vi "JetStages_GUI.vi"(10 "stop 2":refnum<vi>, 11 "GUI_cluster":T1={"Sub Panel"=refnum, "GUIdevice"="Bella_LP_Mode", "CtlRef"=refnum, "User Event in"=refnum}) -> ()   [LabVIEW 2020]
uses:
  Shared/GUI_Template/GUI_master/tcp new data cluster.ctl
  Controls/eventtypdef1.ctl
  Shared/GUI_Template/GUI_master/tcp_new_data_event.ctl
  Controls/GUI_cluster.ctl
panel:
  in  "stepsize::1":dbl=0.02 caption="stepsize" min=0.001 max=1.0
  in  "relativeMove.Axis 2neg::1":bool caption="+Y"
  in  "relativeMove.Axis 1neg::1":bool caption="-X"
  in  "relativeMove.Axis 2pos::1":bool caption="-Y"
  in  "relativeMove.Axis 1pos::1":bool caption="+X"
  in  "relativeMove.Axis 3neg::1":bool caption="-Z"
  in  "relativeMove.Axis 3pos::1":bool caption="+Z"
  in  "Status.Axis 3::1":u16(ring)=3 caption="Status" items=["Not referenced", "Homing", "Moving", "Ready"]
  in  "Position.Axis 3::1":dbl caption="Z" min=-12.0 max=12.0 format="%_4f"
  in  "Status.Axis 2::1":u16(ring)=3 caption="Status" items=["Not referenced", "Homing", "Moving", "Ready"]
  in  "Status.Axis 1::1":u16(ring)=3 items=["Not referenced", "Homing", "Moving", "Ready"]
  in  "Position.Axis 2::1":dbl caption="Y" min=-12.0 max=12.0 format="%_4f"
  in  "Position.Axis 1::1":dbl caption="X" min=-12.0 max=12.0 format="%_4f"
  in  "stop":bool
  out "tcp data event":T2
  out "GUIdevice 1":string="StagingHexapodPI"
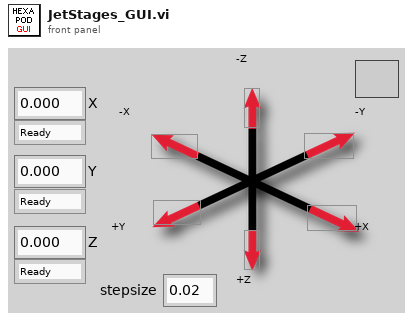
[diagram p1: front panel]
types:
  T1 = typedef "GUI_cluster.ctl" = cluster{"Sub Panel":refnum<vi>, "GUIdevice":string, "CtlRef":refnum<vi>, "User Event in":refnum<user-event>}
  T2 = typedef "tcp_new_data_event.ctl" = refnum<user-event>
  T3 = typedef "eventtypdef1.ctl" = cluster{"label":string, "Sub Panel":refnum<vi>, "CtlRef":refnum<vi>, "This VI":refnum<vi>}
  T4 = typedef "tcp new data cluster.ctl" = cluster{"EventEnum":enum16{"new data", "connection status update"}, "Device name":string}
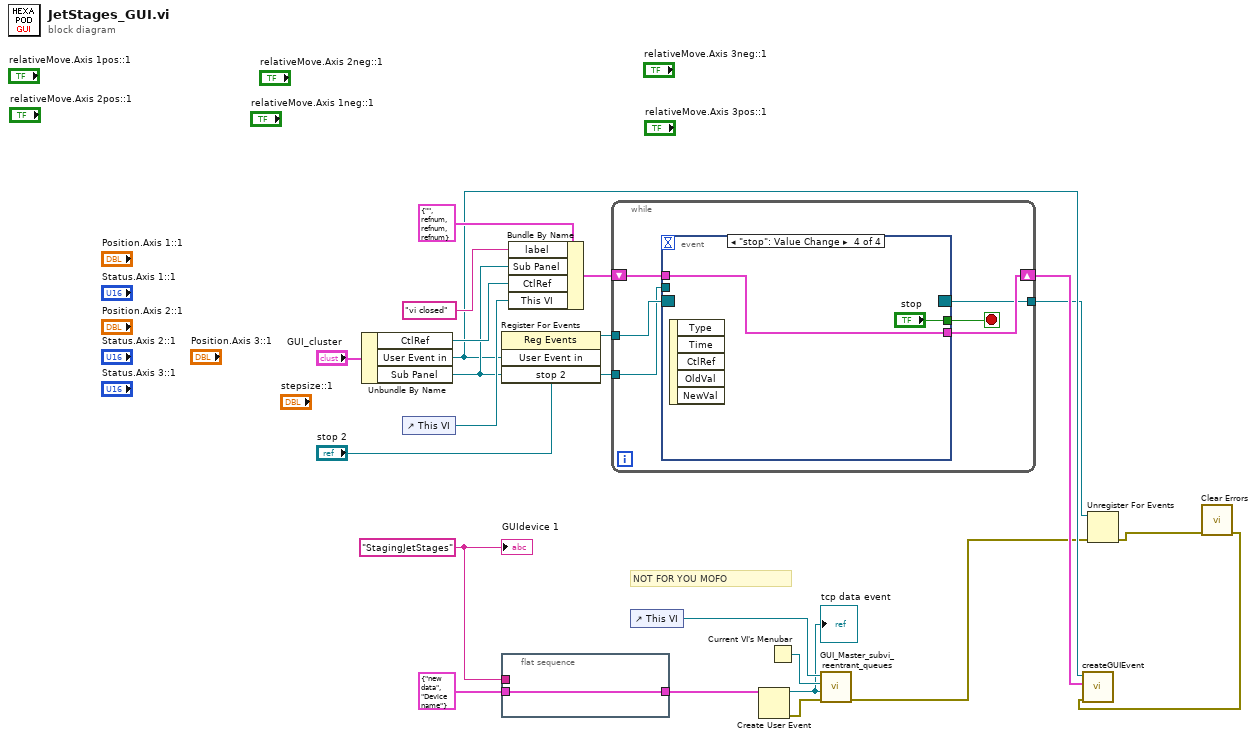
[diagram p0: block diagram]
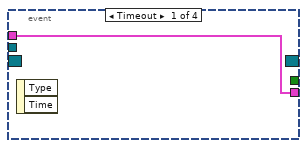
[diagram p2: hidden frame]
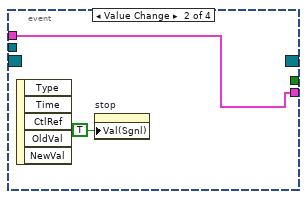
[diagram p3: hidden frame]
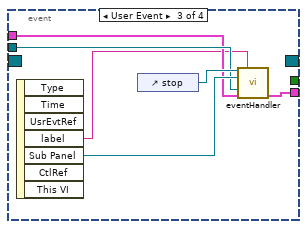
[diagram p4: hidden frame]
diagram:
  w12 = "StagingJetStages" ("GUIdevice")
  # "NOT FOR YOU MOFO"
  n1 = Unbundle By Name("GUI_cluster") -> ("CtlRef"=w14:refnum<vi>, "User Event in"=w7:refnum<user-event>, "Sub Panel"=w9:refnum<vi>)
  n2 = control-ref of="This VI"() -> (w13:refnum<vi>)
  n3 = register-events(w7, "stop 2") -> (reference out=w11:refnum<event-registration>)  [unwired: 2 in, 1 out]
  n4 = flat-sequence {
    tunnel: T4 {"EventEnum"=enum."new data", "Device name"="Device name"} ("New Event") -> [w23]
    tunnel: [w23] -> w15
    tunnel: w12 -> [_]
    frame #0 {
    }
  }
  n5 = Bundle By Name(cluster=T3 {"label"="", "Sub Panel"=refnum, "CtlRef"=refnum, "This VI"=refnum} ("event data"), "label"="vi closed", "Sub Panel"=w9, "CtlRef"=w14, "This VI"=w13) -> (w8:T3)
  n6 = while {
    tunnel: w11 -> [w29]
    tunnel: w9 -> [w27]
    shift-right: [w25] -> w6
    shift-left: w8 -> [w26]
    tunnel: [w24] -> w3
    stop <- w28 stop-if-true
    n7 = event shown="[3] \"stop\": Value Change" {
      selector: w29 -> [_ _ _ _]
      dyn-events: [_ _ _ _] -> w24
      timeout: _ -> [_ _ _ _]
      tunnel: [_ _ _ "stop"] -> w28
      tunnel: w27 -> [_ _ w36 _]
      tunnel: w26 -> [w30 w32 w35 w39]
      tunnel: [w30 w32 w34 w39] -> w25
      event Timeout {
        n8 = event-data() -> ()  [unwired: 1 in, 2 out]
      }
      event Value Change {
        n9 = event-data() -> ()  [unwired: 1 in, 5 out]
        n10 = property on="stop" class="Bool (strict)"("Val(Sgnl)"=TRUE ("Value (Signaling)")) -> ()  [unwired: 2 in, 2 out]
      }
      event User Event {
        n11 = event-data() -> ("label"=w33:string, "Sub Panel"=w37:refnum<vi>)  [unwired: 1 in, 5 out]
        n12 = control-ref of="stop"() -> (w38:refnum<vi>)
        n13 = call "eventHandler.vi"("Boolean in"=w38, "label"=w33, "Sub Panel 2"=w37, "Sub Panel"=w36, "event data in"=w35) -> ("event data out"=w34:T3)  [unwired: 10 in]
      }
      event "stop": Value Change {
        n14 = event-data() -> ()  [unwired: 1 in, 5 out]
      }
    }
  }
  n15 = control-ref of="This VI"() -> (w22:refnum<vi>)
  n16 = Create User Event(user event datatype=w15) -> (user event=w19:refnum<user-event>, error out=w20:errorcluster)  [unwired: 1 in]
  "tcp data event" <- w19
  n17 = Current VI's Menubar() -> (w21:refnum<k9>)
  n18 = call "GUI_Master_subvi_reentrant_queues.vi"("error in (no error)"=w20, "tcp data event"=w19, "Caller menu reference"=w21, "Caller VI ref"=w22) -> ("error out"=w2:errorcluster)  [unwired: 7 in]
  n19 = Unregister For Events(event registration refnum=w3, error in=w2) -> (error out=w4:errorcluster)
  n20 = call <vilib>:"Clear Errors.vi"("error in (no error)"=w4) -> ("error out"=w1:errorcluster)  [unwired: 5 in, 1 out]
  n21 = call "createGUIEvent.vi"("error in (no error)"=w1, "event data"=w6, "User Event in"=w7) -> ()  [unwired: 8 in, 1 out]
  "GUIdevice 1" <- w12
